vi "MC data Queue FGV.vi"(1 "FGV State Command":T1, 3 "error in (no error)":errorcluster) -> (7 "queue out":refnum<queue>, 10 "error out":errorcluster)   [LabVIEW 2020]
uses:
  templates/Queue Access FGV/Controls/FGV State Command.ctl
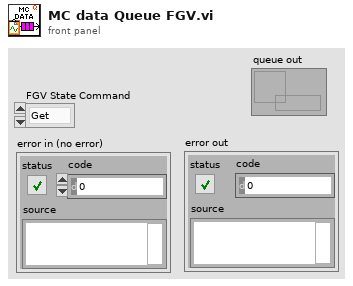
[diagram p1: front panel]
types:
  T1 = typedef "FGV State Command.ctl" = enum16{"Get", "Initialize", "Release"}
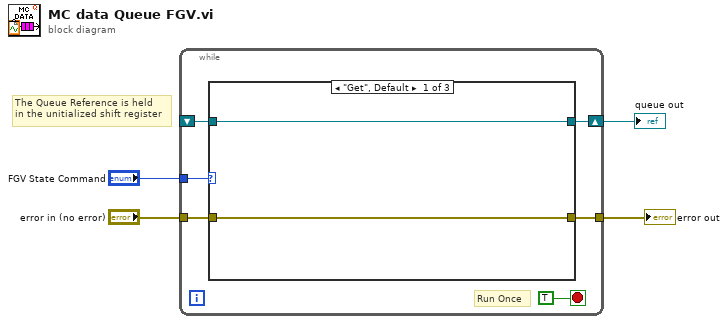
[diagram p0: block diagram]
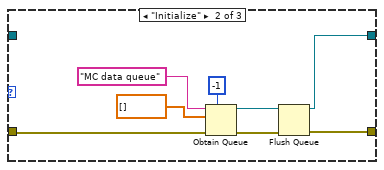
[diagram p2: hidden frame]
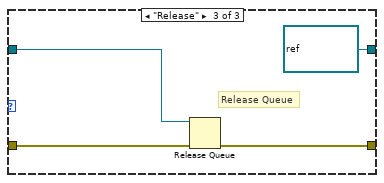
[diagram p3: hidden frame]
diagram:
  # "The Queue Reference is held\nin the unitialized shift register"
  n1 = while {
    tunnel: "FGV State Command" -> [w10]
    shift-right: [w8] -> w1
    shift-left: _ -> [w7]
    tunnel: [w6] -> w2
    tunnel: "error in (no error)" -> [w5]
    stop <- TRUE stop-if-true
    # "Run Once"
    n2 = case shown="\"Get\", Default" w10 {
      tunnel: [w12 w13 refnum<queue> refnum ("queue out")] -> w8
      tunnel: w7 -> [w12 _ w22]
      tunnel: [w11 w14 w23] -> w6
      tunnel: w5 -> [w11 w15 w24]
      frame "Get", Default {
      }
      frame "Initialize" {
        n3 = Obtain Queue(max queue size (-1, unlimited)=-1, name (unnamed)="MC data queue", element data type=dbl[] [], error in (no error)=w15) -> (queue out=w18:refnum<queue>, error out=w17:errorcluster)  [unwired: 1 in, 1 out]
        n4 = Flush Queue(queue=w18, error in (no error)=w17) -> (queue out=w13:refnum<queue>, error out=w14:errorcluster)  [unwired: 1 out]
      }
      frame "Release" {
        # "Release Queue"
        n5 = Release Queue(queue=w22, error in (no error)=w24) -> (error out=w23:errorcluster)  [unwired: 1 in, 2 out]
      }
    }
  }
  "error out" <- w2
  "queue out" <- w1
